vi "Get Array Value at Index - Numeric.vi"(8 "error in (no error)":errorcluster, 9 "Default Value if JSON Null":dbl, 10 "Index":i32, 11 "JSON Tree In (JSON Array)":variant) -> (0 "error out":errorcluster, 1 "is JSON Null?":bool, 2 "Double Value":dbl, 3 "JSON Tree Out Passthrough":variant)   [LabVIEW 2013, in "i3-json.lvlib"]
doc: "Returns the value at a given index from a JSON array"
uses:
  i3-json.lvlib
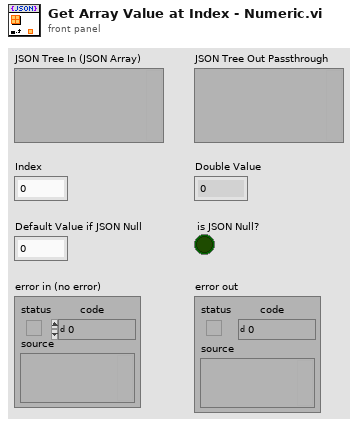
[diagram p1: front panel]
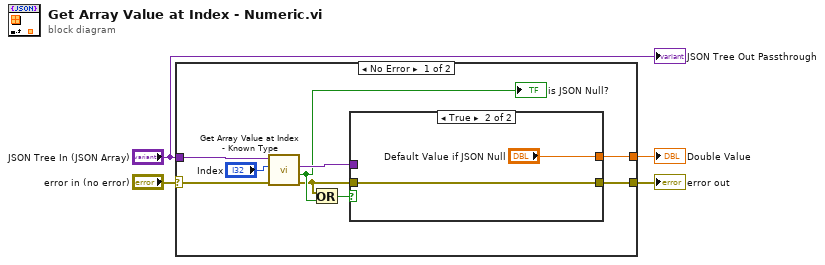
[diagram p0: block diagram]
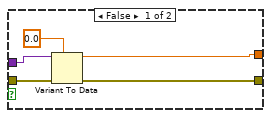
[diagram p2: hidden frame]
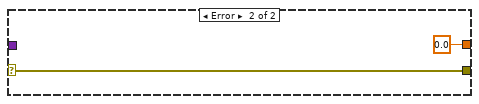
[diagram p3: hidden frame]
diagram:
  n1 = case shown="No Error" "error in (no error)" {
    selector: "error in (no error)" -> [w11 w22]
    tunnel: [w9 w22] -> w3
    tunnel: "JSON Tree In (JSON Array)" -> [w13 _]
    tunnel: [w6 0.0 ("Default Value if JSON Null")] -> w2
    frame No Error {
      n2 = call "Get Array Value at Index - Known Type.vi"("error in (no error)"=w11, "Index"="Index", "JSON Tree In (JSON Array)"=w13) -> ("error out"=w5:errorcluster, "is JSON Null?"=w7:bool, "Value"=w8:variant)  [unwired: 3 in, 3 out]
      "is JSON Null?" <- w7
      n3 = Or(x=w5, y=w7) -> (x .or. y?=w10:bool)
      n4 = case shown="True" w10 {
        tunnel: w5 -> [w18 w20]
        tunnel: [w15 w20] -> w9
        tunnel: w8 -> [w17 _]
        tunnel: [w16 "Default Value if JSON Null"] -> w6
        frame False {
          n5 = Variant To Data(error in=w18, type=0.0 ("Double Value"), Variant=w17) -> (data=w16:dbl, error out=w15:errorcluster)
        }
        frame True {
        }
      }
    }
    frame Error {
    }
  }
  "error out" <- w3
  "Double Value" <- w2
  "JSON Tree Out Passthrough" <- "JSON Tree In (JSON Array)"
